vi "FDMR+ save measurement properties.vi"(7 "FDMR+ script line":T2={"F_start [GHz]"=0.0, "F_end [GHz]"=0.0, "Field [T]"=0.0, "Points [-]"=0, "Sampling Rate"=15, "ModA [G]"=0.0, "ModF [kHz]"=0.0, "Time const [ms]"=10.0, "Angle [°]"=3.0, "Tmp [K]"=0.0, "Wait [min]"=100.0, "Repeat [-]"=1048576, "Comment"="", "Execute"=FALSE, "Auto-mod"=FALSE} {"Sampling Rate" items=["117 ks/S"=9, "58.6 kS/s"=10, "29.3 kS/s"=11, "14.6 kS/s"=12, "7.32 kS/s"=13, "3.66 kS/s"=14, "1.83 kS/s"=15]; "Time const [ms]" format="%_2e"; "ModF [kHz]" min=0.2 max=120.0; "Repeat [-]" max=1048576; "Tmp [K]" min=-1.0 max=330.0; "Field [T]" min=-16.0 max=16.0}, 8 "error in (no error)":errorcluster, 9 "Description":string, 10 "Sample holder":T1, 11 "Refnum in":refnum<k34>) -> (0 "error out":errorcluster, 3 "Refnum out":refnum<k34>)   [LabVIEW 2024]
doc: "Sets a properties of FDMR+ measurement for each channel into TDMS file.\n\nField: Set[T], Unit\nModulation: Frequency[kHz], Set[G], FilterConst[ms], Unit\nVTI: Set[K], Unit\nX sum: SampleHolder, Repeat, Wait[min], FStart[GHz], FEnd[GHz], SweepTime[s], ImF[MHz], Unit\nAngle: Set[°], Unit"
uses:
  Datatypes/FDMR+ script line.ctl
  Subsystem modules/Lock-in module/ctl/OSC sampling rate.ctl
  Datatypes/SampleHolders.ctl
  <vilib>/Analysis/1siggen.llb/Ramp Pattern by Samples.vi
  <vilib>/Analysis/NI_AALBase.lvlib
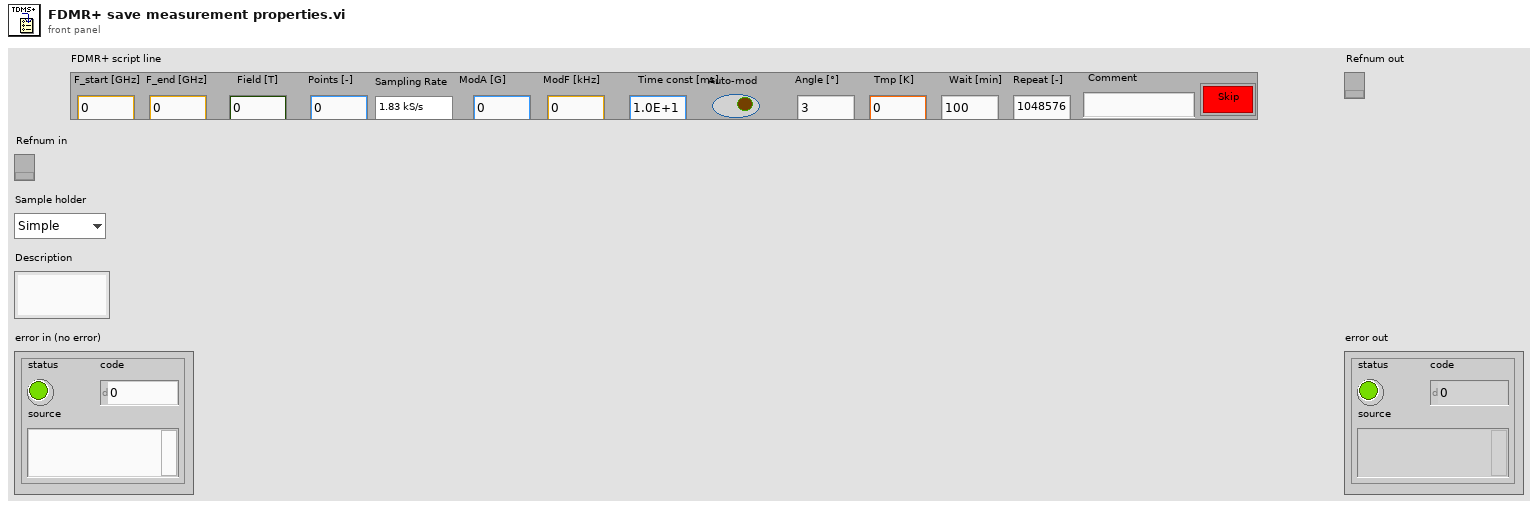
[diagram p1: front panel]
types:
  T1 = typedef "SampleHolders.ctl" = enum16{"Simple", "Carousel", "Chip", "Rotator", "Liquid"}
  T2 = typedef "FDMR+ script line.ctl" = cluster{"F_start [GHz]":dbl, "F_end [GHz]":dbl, "Field [T]":dbl, "Points [-]":u32, "Sampling Rate":T3, "ModA [G]":dbl, "ModF [kHz]":dbl, "Time const [ms]":dbl, "Angle [°]":dbl, "Tmp [K]":dbl, "Wait [min]":dbl, "Repeat [-]":i32, "Comment":string, "Execute":bool, "Auto-mod":bool}
  T3 = typedef "OSC sampling rate.ctl" = u16
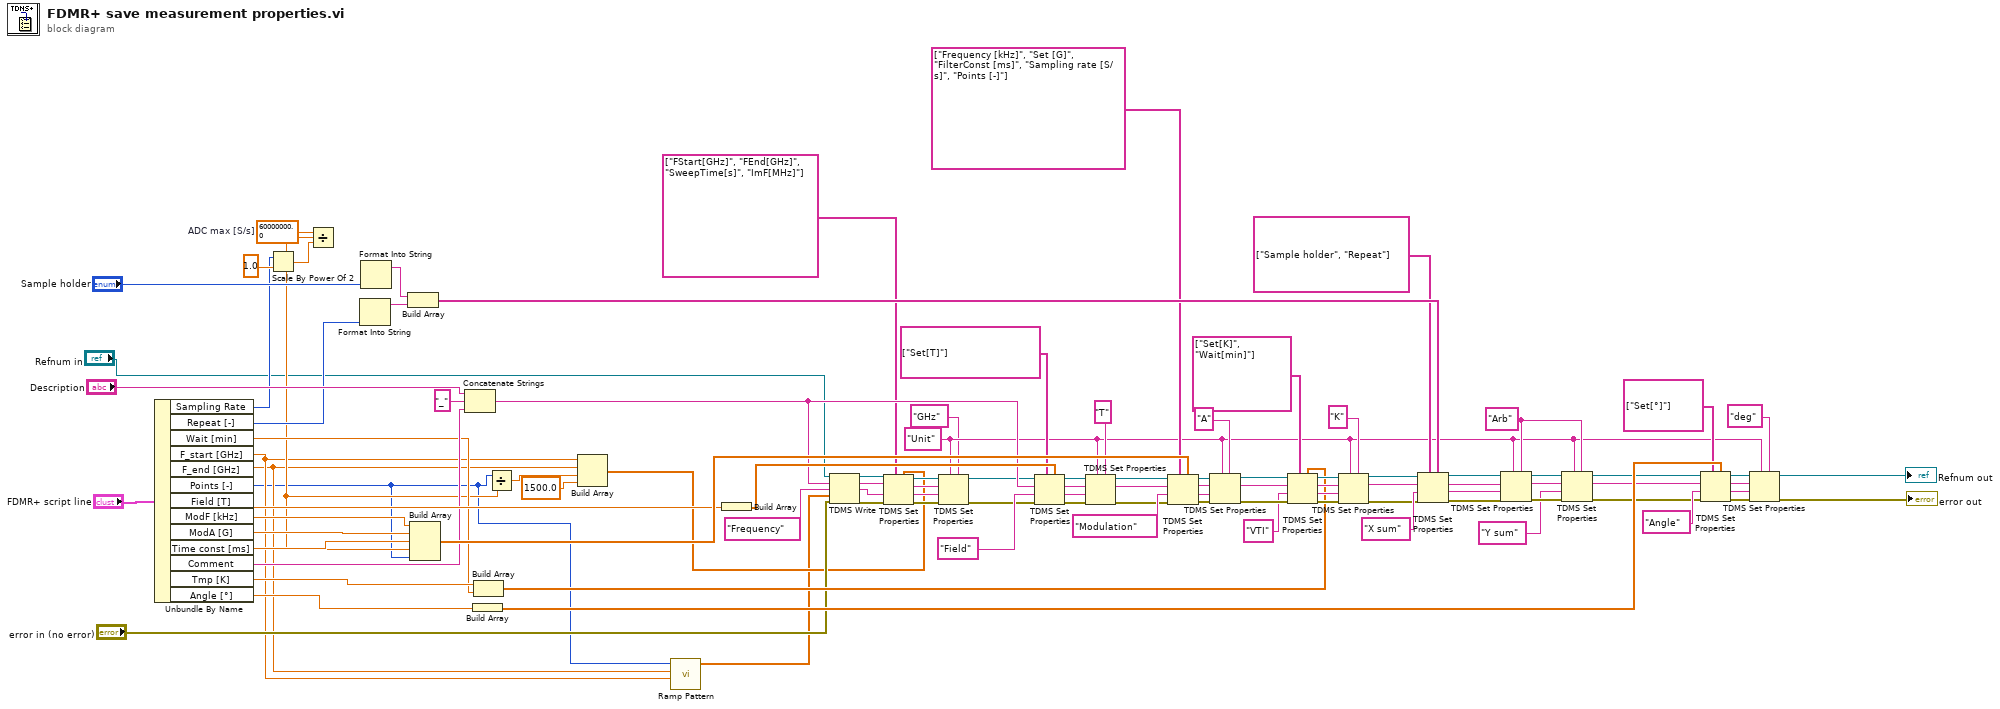
[diagram p0: block diagram]
diagram:
  w33 = 60000000.0  # ADC max [S/s]
  w34 = "Arb"
  w10 = "Unit" ("channel name")
  n1 = Unbundle By Name("FDMR+ script line") -> ("Sampling Rate"=w30:T3, "Repeat [-]"=w43:i32, "Wait [min]"=w42:dbl, "F_start [GHz]"=w9:dbl, "F_end [GHz]"=w8:dbl, "Points [-]"=w7:u32, "Field [T]"=w94:dbl, "ModF [kHz]"=w100:dbl, "ModA [G]"=w101:dbl, "Time const [ms]"=w102:dbl, "Comment"=w78:string, "Tmp [K]"=w56:dbl, "Angle [°]"=w47:dbl)
  n2 = Scale By Power Of 2(n=w30, x=1.0) -> (x*2^n=w32:dbl)
  n3 = Divide(x=w33, y=w32) -> (x/y=w29:dbl)
  n4 = Format Into String(w43) -> (resulting string=w98:string)  [unwired: 3 in, 1 out]
  n5 = Format Into String("Sample holder") -> (resulting string=w86:string)  [unwired: 3 in, 1 out]
  n6 = Build Array(w86, w98) -> (w99:string[])
  n7 = Build Array(w100, w101, w102, w29, w7) -> (w96:dbl[])
  n8 = Concatenate Strings("Description", "_", w78) -> (w23:string)
  n9 = Build Array(w47) -> (w46:dbl[])
  n10 = Build Array(w56, w42) -> (w55:dbl[])
  n11 = Divide(x=w7, y=w29) -> (x/y=w28:dbl)
  n12 = Build Array(w9, w8, w28, 1500.0 ("input 4")) -> (w11:dbl[])
  n13 = call-poly <vilib>:"Ramp Pattern.vi"("start"=w9, "end"=w8, "samples"=w7) -> ("Ramp Pattern"=w6:dbl[])  [unwired: 7 in, 1 out]
  n14 = Build Array(w94) -> (w95:dbl[])
  n15 = TDMS Write(0:"Refnum in", 5:w23, 7:"Frequency", 9:w6, 11:"error in (no error)") -> (4:w18:refnum<k34>, 6:w14:string, 8:w15:string, 15:w22:errorcluster)  [unwired: 1 in]
  n16 = TDMS Set Properties(5:w11, 7:string[] ["FStart[GHz]", "FEnd[GHz]", "SweepTime[s]", "ImF[MHz]"], 8:w22, 9:w15, 10:w14, 11:w18) -> (0:w26:errorcluster, 1:w27:string, 2:w13:string, 3:w17:refnum<k34>)
  n17 = TDMS Set Properties(5:"GHz", 7:w10, 8:w26, 9:w27, 10:w13, 11:w17) -> (0:w21:errorcluster, 3:w16:refnum<k34>)  [unwired: 2 out]
  n18 = TDMS Set Properties(5:w95, 7:string[] ["Set[T]"], 8:w21, 9:"Field", 10:w23, 11:w16) -> (0:w83:errorcluster, 1:w82:string, 2:w81:string, 3:w80:refnum<k34>)
  n19 = TDMS Set Properties(5:"T", 7:w10, 8:w83, 9:w82, 10:w81, 11:w80) -> (0:w75:errorcluster, 2:w77:string, 3:w76:refnum<k34>)  [unwired: 1 out]
  n20 = TDMS Set Properties(5:w96, 7:string[] ["Frequency [kHz]", "Set [G]", "FilterConst [ms]", "Sampling rate [S/s]", "Points [-]"], 8:w75, 9:"Modulation" ("channel name"), 10:w77, 11:w76) -> (0:w71:errorcluster, 1:w72:string, 2:w74:string, 3:w73:refnum<k34>)
  n21 = TDMS Set Properties(5:"A", 7:w10, 8:w71, 9:w72, 10:w74, 11:w73) -> (0:w69:errorcluster, 2:w60:string, 3:w68:refnum<k34>)  [unwired: 1 out]
  n22 = TDMS Set Properties(5:w55, 7:string[] ["Set[K]", "Wait[min]"], 8:w69, 9:"VTI" ("channel name"), 10:w60, 11:w68) -> (0:w67:errorcluster, 1:w66:string, 2:w65:string, 3:w64:refnum<k34>)
  n23 = TDMS Set Properties(5:"K", 7:w10, 8:w67, 9:w66, 10:w65, 11:w64) -> (0:w61:errorcluster, 2:w62:string, 3:w63:refnum<k34>)  [unwired: 1 out]
  n24 = TDMS Set Properties(5:w99, 7:string[] ["Sample holder", "Repeat"], 8:w61, 9:"X sum" ("channel name"), 10:w62, 11:w63) -> (0:w1:errorcluster, 1:w2:string, 2:w3:string, 3:w4:refnum<k34>)
  n25 = TDMS Set Properties(5:w34, 7:w10, 8:w1, 9:w2, 10:w3, 11:w4) -> (0:w40:errorcluster, 2:w36:string, 3:w41:refnum<k34>)  [unwired: 1 out]
  n26 = TDMS Set Properties(5:w34, 7:w10, 8:w40, 9:"Y sum" ("channel name"), 10:w36, 11:w41) -> (0:w39:errorcluster, 2:w37:string, 3:w38:refnum<k34>)  [unwired: 1 out]
  n27 = TDMS Set Properties(5:w46, 7:string[] ["Set[°]"], 8:w39, 9:"Angle" ("channel name"), 10:w37, 11:w38) -> (0:w51:errorcluster, 1:w48:string, 2:w49:string, 3:w53:refnum<k34>)
  n28 = TDMS Set Properties(5:"deg", 7:w10, 8:w51, 9:w48, 10:w49, 11:w53) -> (0:→"error out":errorcluster, 3:→"Refnum out":refnum<k34>)  [unwired: 2 out]
